vi "File.Move_Copy File, Overwrite if Exists.vi"(6 "Move(F)/Copy(T)":bool, 7 "SkipIfExists(F)/Overwrite(T)":bool=TRUE, 8 "error in":errorcluster, 10 "Target Path":path, 11 "Source Path":path) -> (0 "error out":errorcluster, 3 "Target Out":path)   [LabVIEW 2019]
uses:
  <vilib>/KATE/Files/File Utils.lvlib
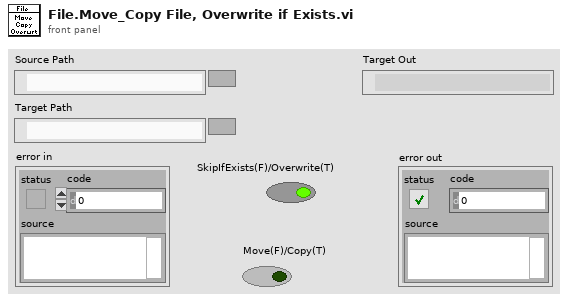
[diagram p1: front panel]
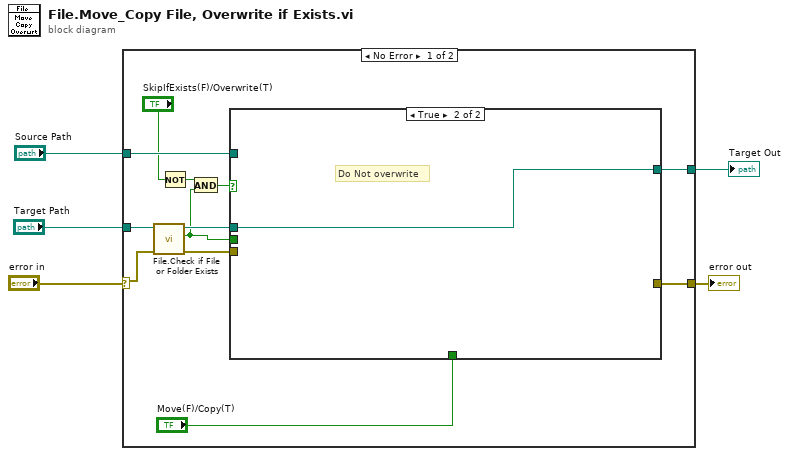
[diagram p0: block diagram]
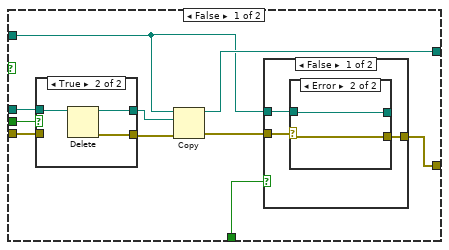
[diagram p2: hidden frame]
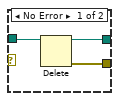
[diagram p3: hidden frame]
diagram:
  n1 = case shown="No Error" "error in" {
    selector: "error in" -> [w14 w43]
    tunnel: "Target Path" -> [w16 w42]
    tunnel: [w11 w43] -> w4
    tunnel: "Source Path" -> [w12 _]
    tunnel: [w13 w42] -> w1
    frame No Error {
      n2 = call <vilib>:"File.Check if File or Folder Exists.vi"("error in"=w14, "Path"=w16) -> ("error out"=w15:errorcluster, "Exists"=w8:bool, "Dup Path"=w17:path)  [unwired: 5 in, 2 out]
      n3 = Not(x="SkipIfExists(F)/Overwrite(T)") -> (.not. x?=w7:bool)
      n4 = And(x=w7, y=w8) -> (x .and. y?=w9:bool)
      n5 = case shown="True" w9 {
        tunnel: w8 -> [w27 _]
        tunnel: w17 -> [w26 w41]
        tunnel: w15 -> [w25 _]
        tunnel: [w22 w41] -> w13
        tunnel: w12 -> [w21 _]
        tunnel: [w19 _] -> w11
        tunnel: "Move(F)/Copy(T)" -> [w18 _]
        frame False {
          n6 = case shown="True" w27 {
            tunnel: w26 -> [w37 w40]
            tunnel: [_ w39] -> w23
            tunnel: [w37 w38] -> w24
            tunnel: w25 -> [_ _]
            frame False {
            }
            frame True {
              n7 = Delete(path (use dialog)=w40) -> (deleted path=w38:path, error out=w39:errorcluster)  [unwired: 4 in, 1 out]
            }
          }
          n8 = Copy(8:w23, 10:w24, 11:w21) -> (0:w20:errorcluster, 3:w22:path)  [unwired: 2 in, 1 out]
          n9 = case shown="False" w18 {
            tunnel: w21 -> [w30 _]
            tunnel: w20 -> [w29 w36]
            tunnel: [w28 w36] -> w19
            frame False {
              n10 = case shown="Error" w29 {
                selector: w29 -> [_ w34]
                tunnel: w30 -> [w33 w35]
                tunnel: [w32 w34] -> w28
                tunnel: [w31 w35] -> _
                frame No Error {
                  n11 = Delete(path (use dialog)=w33) -> (deleted path=w31:path, error out=w32:errorcluster)  [unwired: 4 in, 1 out]
                }
                frame Error {
                }
              }
            }
            frame True {
            }
          }
        }
        frame True {
          # "Do Not overwrite"
        }
      }
    }
    frame Error {
    }
  }
  "error out" <- w4
  "Target Out" <- w1
